vi "Day 2-2.vi"() -> ()   [LabVIEW 2019, in "Day 2.lvlib"]
uses:
  <vilib>/Utility/error.llb/Error Cluster From Error Code.vi
  <vilib>/ErrorRing/Error Ring.xnode
  Day 2.lvlib
panel:
  out "Array 2":bool[][](array[boolean])
  out "error IO":errorcluster
  out "Array":string[](array[string])
  in  "String":string="010110011101\n101100111000\n100100000011\n111000010001\n001100010011\n010000111100\n001000100011\n001000100111\n010001111110\n111101001011\n011000101011\n111100111001\n100101111011\n101100110110\n101010111001\n001111000110\n001001101000\n101011001010\n011101111010\n011101001010\n011001000001\n100001010000\n111011001101\n000111110111\n010011001111\n000111011001\n111000010100\n101001100100\n110010001101\n111110101000\n011001100010\n110010110101\n010000001101\n100000000100\n110111011110\n110001100110\n001011110111\n110000011110\n110110101010\n101001100110\n010000001010\n100010100100\n101000111101\n111000001011\n000000100100\n100111010110\n01..."
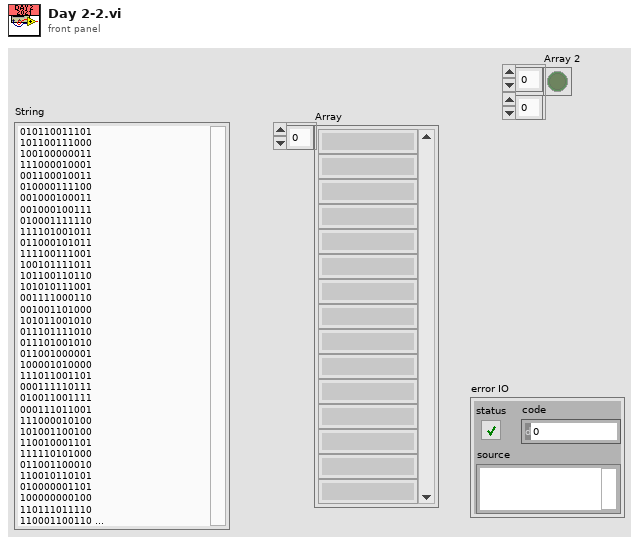
[diagram p1: front panel]
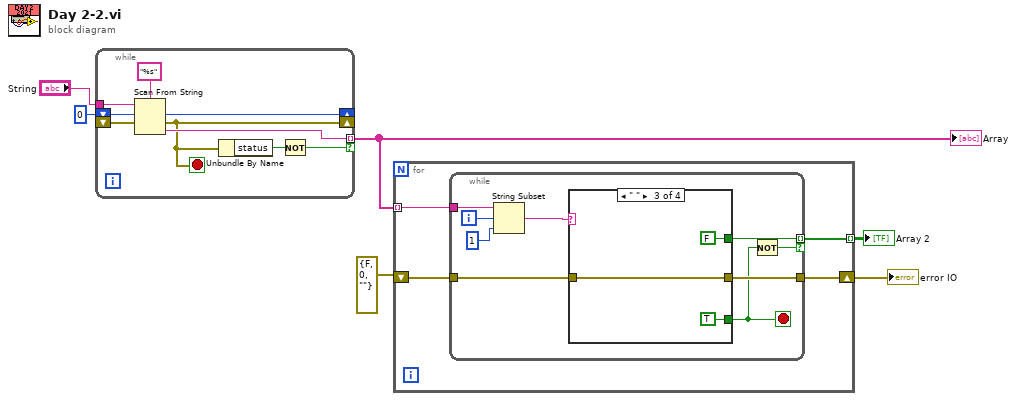
[diagram p0: block diagram]
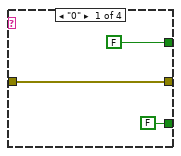
[diagram p2: hidden frame]
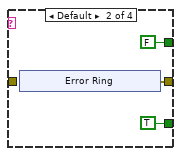
[diagram p3: hidden frame]
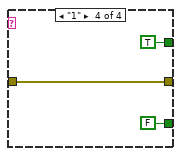
[diagram p4: hidden frame]
diagram:
  n1 = while {
    tunnel: [w13] -> w4 mode=indexing if=w7
    tunnel: "String" -> [w15]
    shift-right: [w10] -> _
    shift-left: u32 0 -> [w12]
    shift-right: [w9] -> _
    shift-left: _ -> [w11]
    stop <- w9 stop-if-true
    n2 = Scan From String(format string="%s", input string=w15, initial scan location=w12, error in=w11) -> (offset past scan=w10:u32, error out=w9:errorcluster, output 1=w13:string)  [unwired: 1 in, 1 out]
    n3 = Unbundle By Name(w9) -> ("status"=w8:bool)
    n4 = Not(x=w8) -> (.not. x?=w7:bool)
  }
  "Array" <- w4
  n5 = for {
    tunnel: w4 -> [w19] mode=indexing
    shift-right: [w16] -> w3
    shift-left: errorcluster {"status"=FALSE, "code"=0, "source"=""} ("error out") -> [w18]
    tunnel: [w17] -> w1 mode=indexing
    n6 = while {
      tunnel: w19 -> [w28]
      tunnel: w18 -> [w24]
      tunnel: [w23] -> w17 mode=indexing if=w21
      tunnel: [w22] -> w16
      i -> [w27]
      stop <- w20 stop-if-true
      n7 = String Subset(string=w28, offset (0)=w27, length (rest)=1 ("length (rest)")) -> (substring=w25:string)
      n8 = case shown="\" \"" w25 {
        tunnel: [w31 w34 w42 w45] -> w22
        tunnel: w24 -> [w31 _ w42 w45]
        tunnel: [FALSE FALSE FALSE TRUE] -> w23
        tunnel: [FALSE TRUE TRUE FALSE] -> w20
        frame "0" {
        }
        frame Default {
          n9 = xnode "Error Ring"() -> ("error out"=w34:errorcluster)
        }
        frame " " {
        }
        frame "1" {
        }
      }
      n10 = Not(x=w20) -> (.not. x?=w21:bool)
    }
  }
  "error IO" <- w3
  "Array 2" <- w1
